vi "ProgramPowerBoard.vi"(11 "BitstreamFilename":string) -> (3 "return code":i32)   [LabVIEW 2009]
panel:
  out "UseImpactErrorOut":errorcluster
  out "CreateBatchFileErrorOut":errorcluster
  out "standard output":string
  out "standard error":string
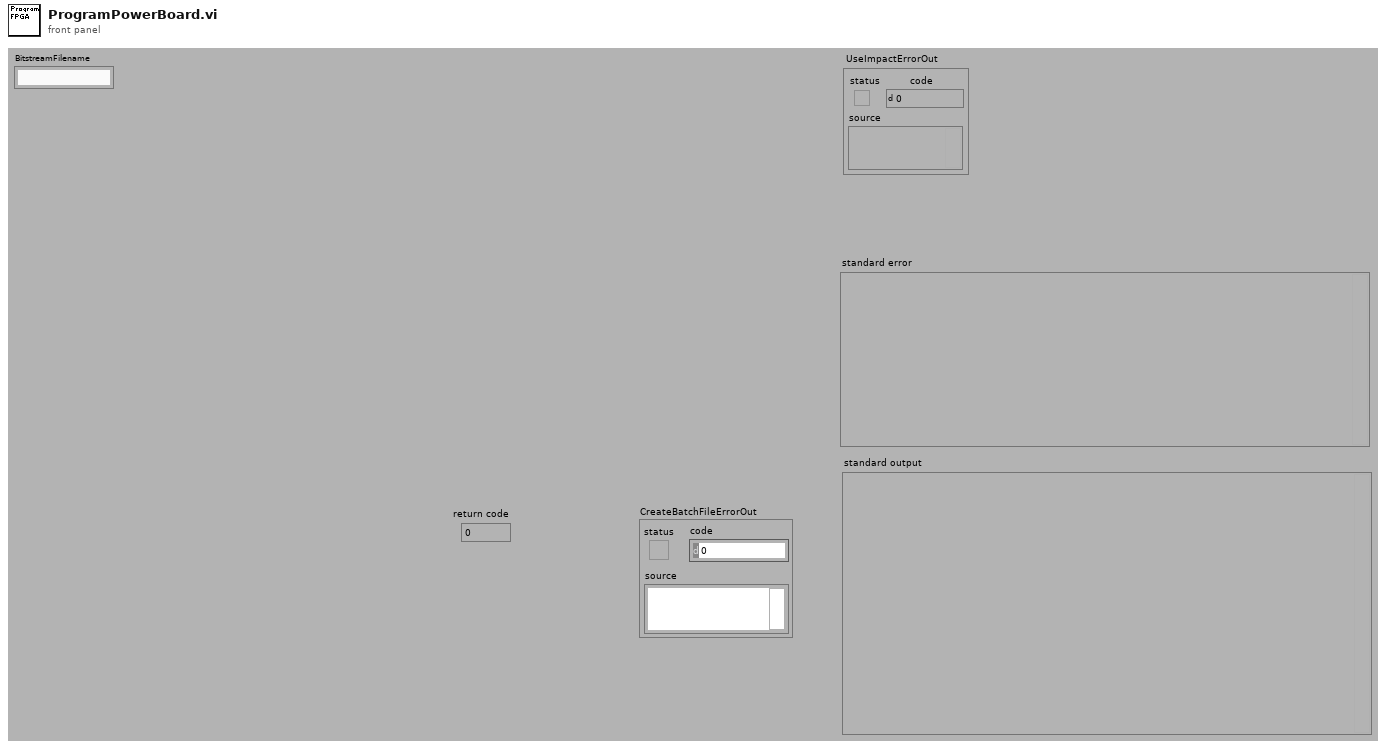
[diagram p1: front panel]
types:
  T1 = enum16{"open", "replace", "create", "open or create", "replace or create", "replace or create with confirmation"}
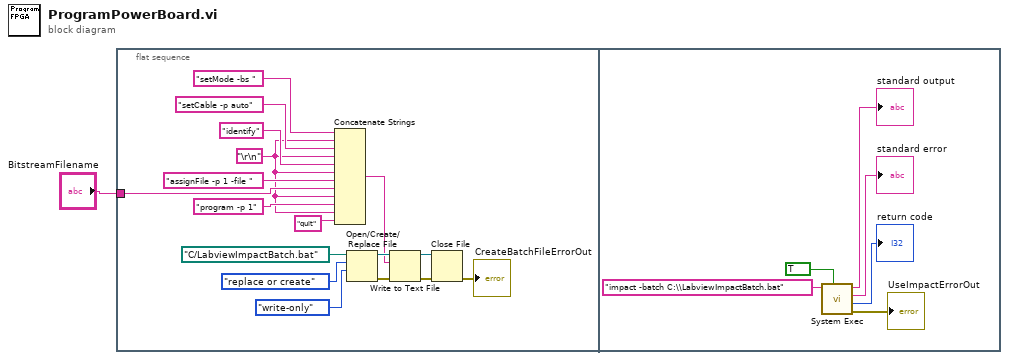
[diagram p0: block diagram]
diagram:
  n1 = flat-sequence {
    tunnel: "BitstreamFilename" -> [w6]
    frame #0 {
      w4 = "\r\n"
      n2 = Concatenate Strings("setMode -bs " ("string"), w4, "setCable -p auto" ("string"), w4, "identify" ("string"), w4, "assignFile -p 1 -file " ("string"), w6, w4, "program -p 1" ("string"), w4, "quit" ("string")) -> (w2:string)
      n3 = Open/Create/Replace File(file path (use dialog)=path "C:/LabviewImpactBatch.bat", operation (0:open)=T1."replace or create", access (0:read/write)=enum16{"read/write", "read-only", "write-only"}."write-only") -> (refnum out=w17:refnum<file>, error out=w13:errorcluster)  [unwired: 3 in, 1 out]
      n4 = Write to Text File(file (use dialog)=w17, text=w2, error in=w13) -> (refnum out=w18:refnum<file>, error out=w12:errorcluster)  [unwired: 1 in, 1 out]
      n5 = Close File(refnum=w18, error in=w12) -> (error out=→"CreateBatchFileErrorOut":errorcluster)  [unwired: 1 out]
    }
    frame #1 {
      n6 = call <vilib>:"System Exec.vi"("wait until completion? (T)"=TRUE, "command line"="impact -batch C:\\LabviewImpactBatch.bat") -> ("error out"=→"UseImpactErrorOut":errorcluster, "return code"=→"return code":i32, "standard error"=→"standard error":string, "standard output"=→"standard output":string)  [unwired: 6 in]
    }
  }
